vi "dfd_Direct IIR II Normalization.vi"(7 "scale type":T1, 9 "coefficients b":dbl[](array[numeric]) format="%.2f", 10 "coefficients a":dbl[](array[numeric]) format="%.2f", 11 "x":dbl[](array[numeric])) -> (2 "norm":dbl[](array[numeric]) format="%.2f", 3 "y":dbl[](array[numeric]))   [LabVIEW 2017, in "NI_DigFilter_FXP.lvlib"]
uses:
  <vilib>/addons/Digital Filter Design/NI_DigFilter_FXP.lvlib
  <vilib>/addons/Digital Filter Design/_Objects.llb/DFD Coef Norm Type.ctl
  <vilib>/addons/Digital Filter Design/NI_DigFilterLicensed.lvlib
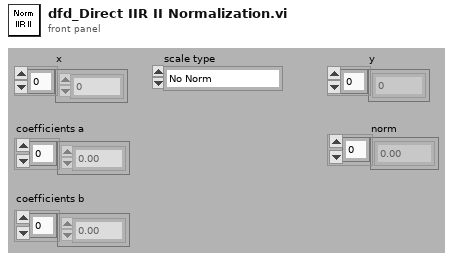
[diagram p1: front panel]
types:
  T1 = typedef "NI_DigFilterLicensed.lvlib/DFD Coef Norm Type.ctl" = enum16{"No Norm", "Time Domain 1-Norm", "Time Domain 2-Norm", "Time Domain Inf-Norm"}
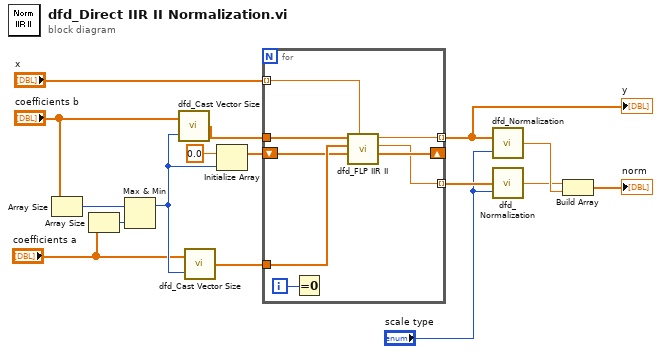
[diagram p0: block diagram]
diagram:
  n1 = Array Size(array="coefficients b") -> (size(s)=w12:i32)
  n2 = Array Size(array="coefficients a") -> (size(s)=w13:i32)
  n3 = Max & Min(x=w12, y=w13) -> (max(x,y)=w6:i32)  [unwired: 1 out]
  n4 = call <vilib>:"dfd_Cast Vector Size.vi"("expected size"=w6, "vector in"="coefficients b") -> ("vector out"=w5:dbl[])
  n5 = call <vilib>:"dfd_Cast Vector Size.vi"("expected size"=w6, "vector in"="coefficients a") -> ("vector out"=w7:dbl[])
  n6 = Initialize Array(0.0 ("element"), w6) -> (w16:dbl[])
  n7 = for {
    shift-right: [w20] -> _
    shift-left: w16 -> [w22]
    tunnel: [w21] -> w1 mode=indexing
    tunnel: w7 -> [w24]
    tunnel: w5 -> [w23]
    tunnel: [w18] -> w11 mode=indexing
    tunnel: "x" -> [w17] mode=indexing
    i -> [w19]
    (unwired) 0.0 ("element")
    n8 = Equal To 0?(x=w19) -> ()  [unwired: 1 out]
    n9 = call <vilib>:"dfd_FLP IIR II.vi"("x"=w17, "states in"=w22, "coefficients a"=w24, "coefficients b"=w23) -> ("states out"=w20:dbl[], "w"=w18:dbl, "y"=w21:dbl)  [unwired: 1 in, 4 out]
  }
  "y" <- w1
  n10 = call <vilib>:"dfd_Normalization.vi"("scale type"="scale type", "h(n)"=w1) -> ("norm"=w10:dbl)
  n11 = call <vilib>:"dfd_Normalization.vi"("scale type"="scale type", "h(n)"=w11) -> ("norm"=w8:dbl)
  n12 = Build Array(w8, w10) -> (→"norm":dbl[])
